vi "Sort Calibration Points.vi"(8 "error in (no error)":errorcluster, 11 "Calibration Points":T1[](array[typedef])) -> (0 "error out":errorcluster, 3 "Sorted Calibration Points":T1[][](array[typedef]))   [LabVIEW 2026, in "Analysis.lvlib"]
uses:
  Analysis.lvlib
  controls/Messaging Payloads/Calibration Point Table Insert.ctl
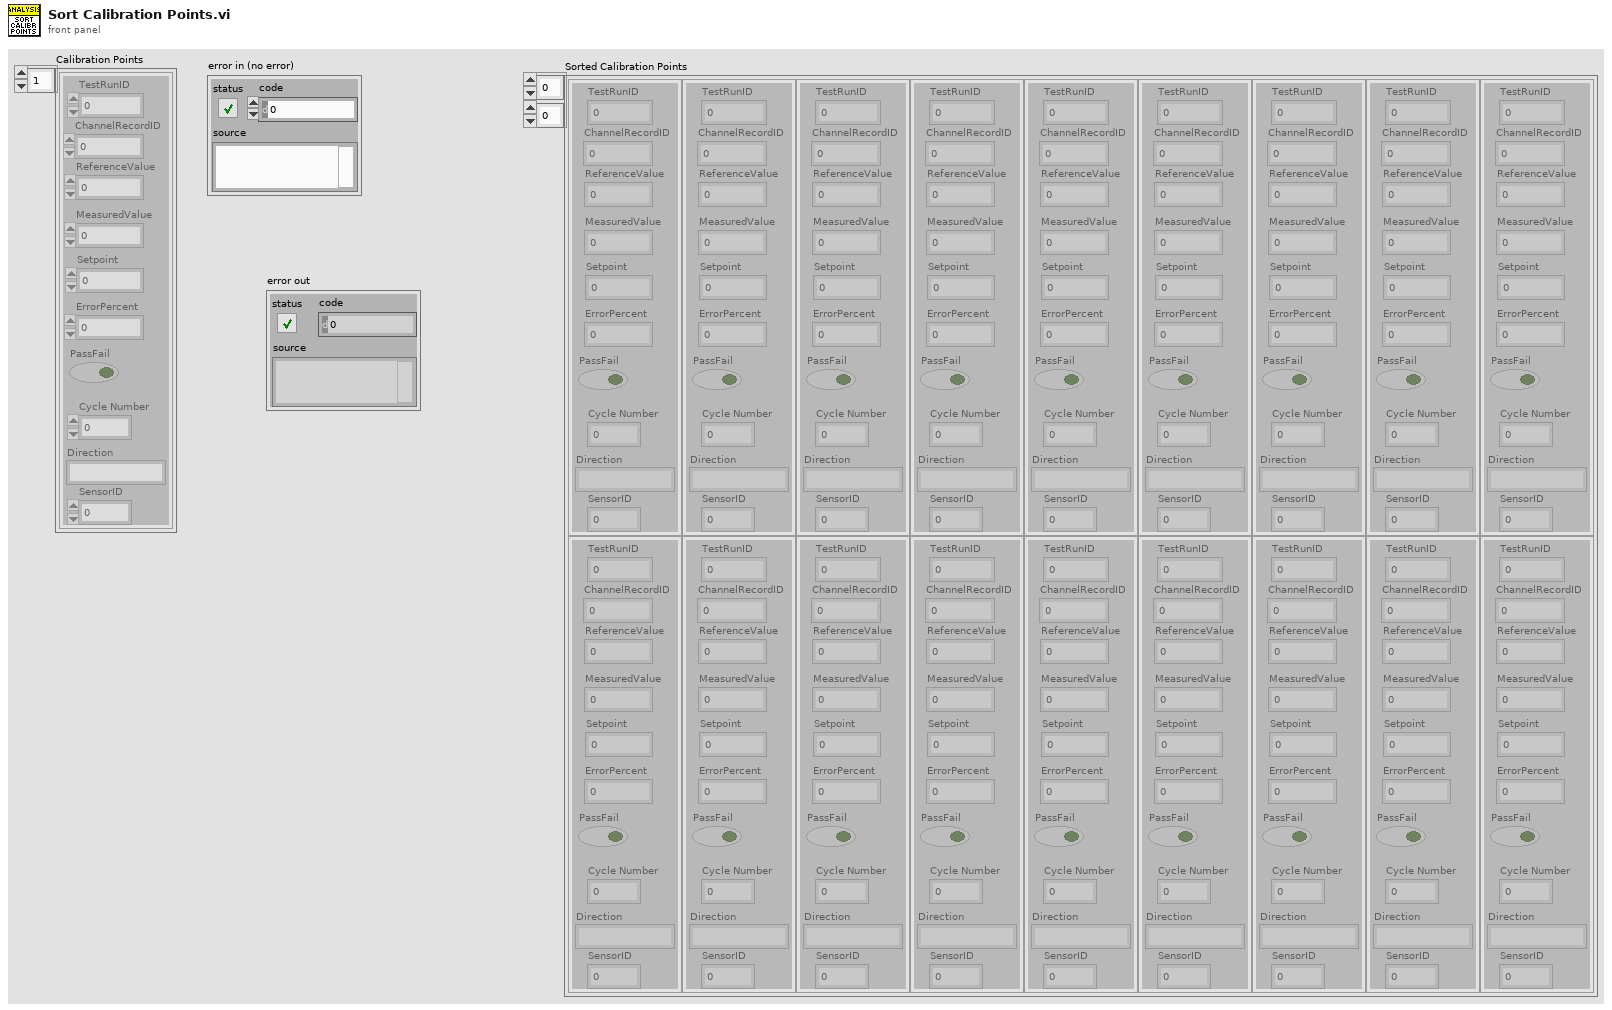
[diagram p1: front panel]
types:
  T1 = typedef "Calibration Point Table Insert.ctl" = cluster{"TestRunID":i32, "ChannelRecordID":i32, "Setpoint":dbl, "MeasuredValue":dbl, "ErrorPercent":dbl, "PassFail":bool, "ReferenceValue":dbl, "Cycle Number":i32, "Direction":string, "SensorID":i32}
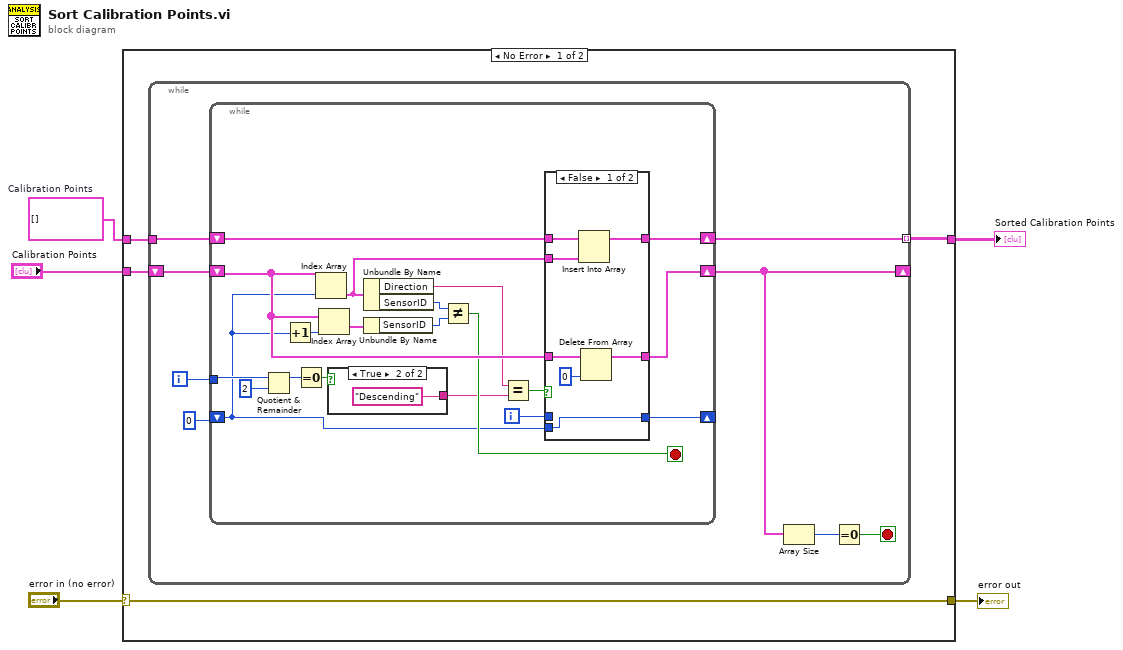
[diagram p0: block diagram]
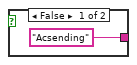
[diagram p2: hidden frame]
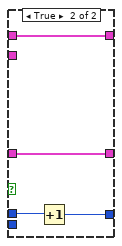
[diagram p3: hidden frame]
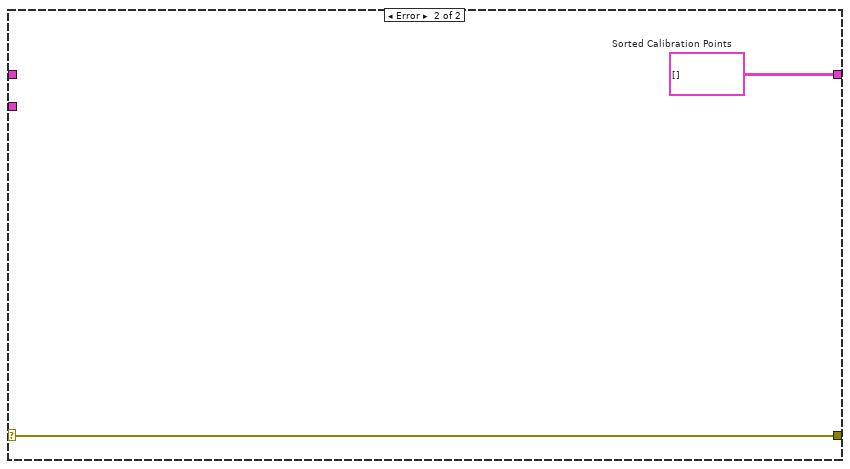
[diagram p4: hidden frame]
diagram:
  w4 = T1[] []  # Calibration Points
  n1 = case shown="No Error" "error in (no error)" {
    selector: "error in (no error)" -> [w7 w52]
    tunnel: "Calibration Points" -> [w9 _]
    tunnel: w4 -> [w8 _]
    tunnel: [w6 w51] -> w3
    tunnel: [w7 w52] -> w1
    frame No Error {
      n2 = while {
        tunnel: w8 -> [w17]
        tunnel: [w16] -> w6 mode=indexing
        shift-right: [w12] -> _
        shift-left: w9 -> [w15]
        i -> [w11]
        stop <- w13 stop-if-true
        n3 = while {
          shift-right: [w37] -> w16
          shift-left: w17 -> [w34]
          shift-right: [w30] -> w12
          shift-left: w15 -> [w32]
          tunnel: w11 -> [w25]
          shift-right: [w20] -> _
          shift-left: 0 -> [w19]
          i -> [w21]
          stop <- w29 stop-if-true
          n4 = Quotient & Remainder(x=w25, y=2) -> (x-y*floor(x/y)=w23:i32)  [unwired: 1 out]
          n5 = Increment(x=w19) -> (x+1=w18:i32)
          n6 = Equal To 0?(x=w23) -> (x = 0?=w22:bool)
          n7 = Index Array(array=w32, index=w19) -> (element=w31:T1)
          n8 = Index Array(array=w32, index=w18) -> (element=w36:T1)
          n9 = case shown="True" w22 {
            tunnel: ["Acsending" "Descending"] -> w27
            frame False {
            }
            frame True {
            }
          }
          n10 = Unbundle By Name(w31) -> ("Direction"=w28:string, "SensorID"=w33:i32)
          n11 = Unbundle By Name(w36) -> ("SensorID"=w35:i32)
          n12 = Not Equal?(x=w33, y=w35) -> (x != y?=w29:bool)
          n13 = Equal?(x=w28, y=w27) -> (x = y?=w26:bool)
          n14 = case shown="False" w26 {
            tunnel: [w46 w49] -> w37
            tunnel: w34 -> [w45 w49]
            tunnel: w32 -> [w44 w50]
            tunnel: w31 -> [w43 _]
            tunnel: [w42 w50] -> w30
            tunnel: w21 -> [_ w48]
            tunnel: [w40 w47] -> w20
            tunnel: w19 -> [w40 _]
            frame False {
              n15 = Insert Into Array(array=w45, new element=w43) -> (w46:T1[])  [unwired: 1 in]
              n16 = Delete From Array(array=w44, index=0) -> (array with subset deleted=w42:T1[])  [unwired: 1 in, 1 out]
            }
            frame True {
              n17 = Increment(x=w48) -> (x+1=w47:i32)
            }
          }
        }
        n18 = Array Size(array=w12) -> (size(s)=w14:i32)
        n19 = Equal To 0?(x=w14) -> (x = 0?=w13:bool)
      }
    }
    frame Error {
      w51 = T1[][] []  # Sorted Calibration Points
    }
  }
  "Sorted Calibration Points" <- w3
  "error out" <- w1
